vi "ActKeyboardAdd.vi"(8 "Error":errorcluster, 9 "Cmd":string, 10 "ChatId":i32, 11 "ActKeyboards in":cluster{"ChatId":i32, "Cmd":string}[](array[cluster])) -> (0 "Error":errorcluster, 3 "ActKeyboards out":cluster{"ChatId":i32, "Cmd":string}[](array[cluster]))   [LabVIEW 2015]
uses:
  Telegram/Methods/TypeDefs/CommandList.ctl
panel:
  out "ActKeyboards out":cluster{"Cmd":T1, "ChatId":i32}[](array[cluster])
  in  "ActKeyboards in":cluster{"Cmd":T1, "ChatId":i32}[](array[cluster])
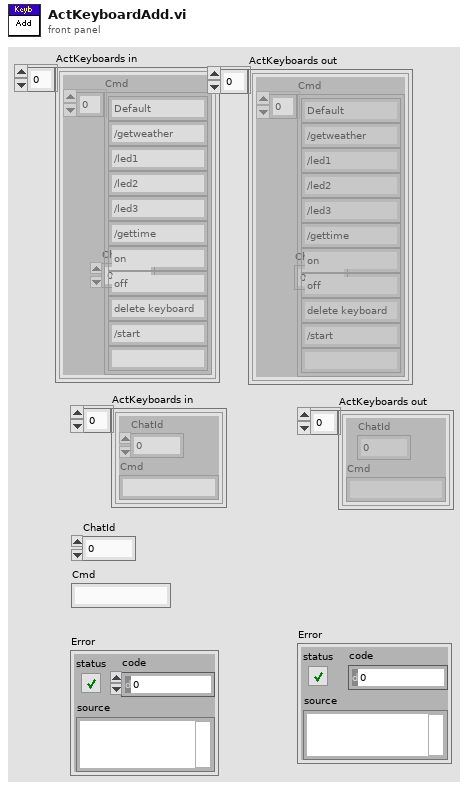
[diagram p1: front panel]
types:
  T1 = typedef "CommandList.ctl" = string[]
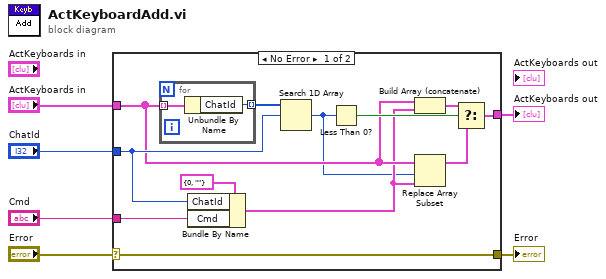
[diagram p0: block diagram]
diagram:
  n1 = case shown="No Error" "Error" {
    selector: "Error" -> [w11 w22]
    tunnel: [w14 w21] -> w2
    tunnel: "ActKeyboards in" -> [w10 w21]
    tunnel: "ChatId" -> [w13 _]
    tunnel: [w11 w22] -> w3
    tunnel: "Cmd" -> [w12 _]
    frame No Error {
      n2 = for {
        tunnel: w10 -> [w20] mode=indexing
        tunnel: [w19] -> w18 mode=indexing
        n3 = Unbundle By Name(w20) -> ("ChatId"=w19:i32)
      }
      n4 = Bundle By Name(cluster=cluster{"ChatId":i32, "Cmd":string} {"ChatId"=0, "Cmd"=""} ("AcriveKeyboard"), "ChatId"=w13, "Cmd"=w12) -> (w9:cluster{"ChatId":i32, "Cmd":string})
      n5 = Search 1D Array(1D array=w18, element=w13) -> (index of element=w8:i32)  [unwired: 1 in]
      n6 = Less Than 0?(x=w8) -> (x < 0?=w17:bool)
      n7 = Build Array (concatenate)(w10, w9) -> (w15:cluster{"ChatId":i32, "Cmd":string}[])
      n8 = Replace Array Subset(array=w10, new element=w9, index=w8) -> (w7:cluster{"ChatId":i32, "Cmd":string}[])
      n9 = Select(t=w15, s=w17, f=w7) -> (s? t:f=w14:cluster{"ChatId":i32, "Cmd":string}[])
    }
    frame Error {
    }
  }
  "Error" <- w3
  "ActKeyboards out" <- w2
